vi "Add Model.vi"(8 "error in (no error)":errorcluster, 10 "OBJ File":path, 11 "Scene in":refnum<class "Scene.lvclass">) -> (0 "error out":errorcluster, 3 "Scene out":refnum<class "Scene.lvclass">)   [LabVIEW 2022 SP3, in "Application.lvlib" / "Scene.lvclass"]
uses:
  Scene.lvclass
  Libraries/3D/Transform.ctl
  Libraries/3D/Vector 3D.ctl
  Scene.lvclass/Scene.ctl
  Libraries/3D/3D.lvlib
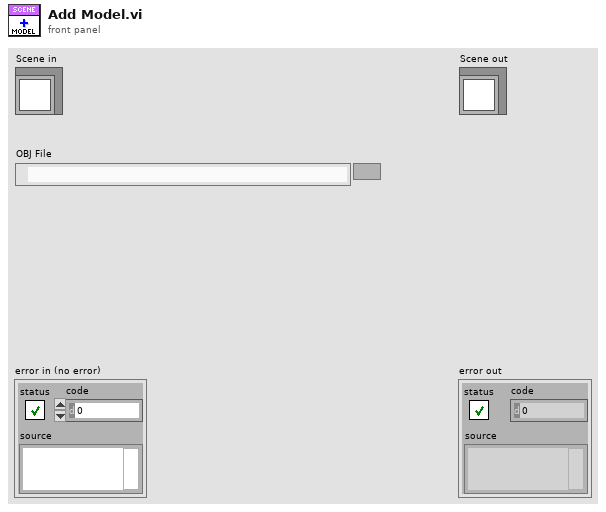
[diagram p1: front panel]
types:
  T1 = typedef "3D.lvlib/Transform.ctl" = cluster{"Position":T2, "Rotation":T2, "Scale":T2}
  T2 = typedef "3D.lvlib/Vector 3D.ctl" = cluster{"x":sgl, "y":sgl, "z":sgl}
  T3 = typedef "3D.lvlib/Object.ctl" = cluster{"Triangles":T4[], "Diffuse Colour":u32, "Transform":T1, "Name":string, "Alpha Blending Enabled":bool, "Alpha":dbl, "Turntable Enabled":bool}
  T4 = typedef "3D.lvlib/Triangle 3D.ctl" = cluster{"Point 1":T2, "Point 2":T2, "Point 3":T2}
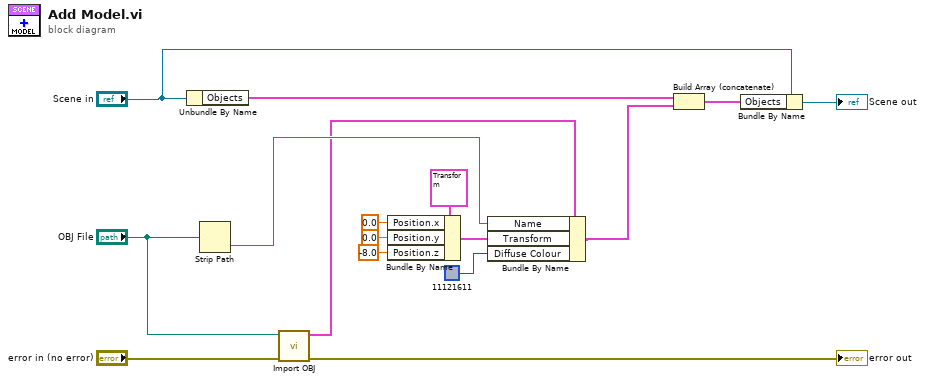
[diagram p0: block diagram]
diagram:
  n1 = Unbundle By Name("Scene in") -> ("Objects"=w9:T3[])
  n2 = Strip Path(path="OBJ File") -> (name=w16:string)  [unwired: 1 out]
  n3 = call "Import OBJ.vi"("error in (no error)"="error in (no error)", "Object"="OBJ File") -> ("error out"=→"error out":errorcluster, "Object"=w2:T3)  [unwired: 8 in]
  n4 = Bundle By Name(cluster=T1 {"Position"={"x"=2.0, "y"=1.0, "z"=-5.0}, "Rotation"={"x"=0.0, "y"=0.0, "z"=0.0}, "Scale"={"x"=0.0, "y"=0.0, "z"=0.0}} ("Transform"), "Position.x"=sgl 0.0, "Position.y"=sgl 0.0, "Position.z"=sgl -8.0) -> (w12:T1)
  n5 = Bundle By Name(cluster=w2, "Name"=w16, "Transform"=w12, "Diffuse Colour"=u32 11121611) -> (w4:T3)
  n6 = Build Array (concatenate)(w9, w4) -> (w5:T3[])
  n7 = Bundle By Name(cluster="Scene in", "Objects"=w5) -> (→"Scene out":refnum<class "Scene.lvclass">)
